vi "mfd_radio_bat.vi"() -> ()   [LabVIEW 2023]
uses:
  <vilib>/Utility/miscctls.llb/LVBoundsTypeDef.ctl
panel:
  in  "MFD_RcControl":T1
  in  "stop":bool
  out "MFD_RadioBattery":picture
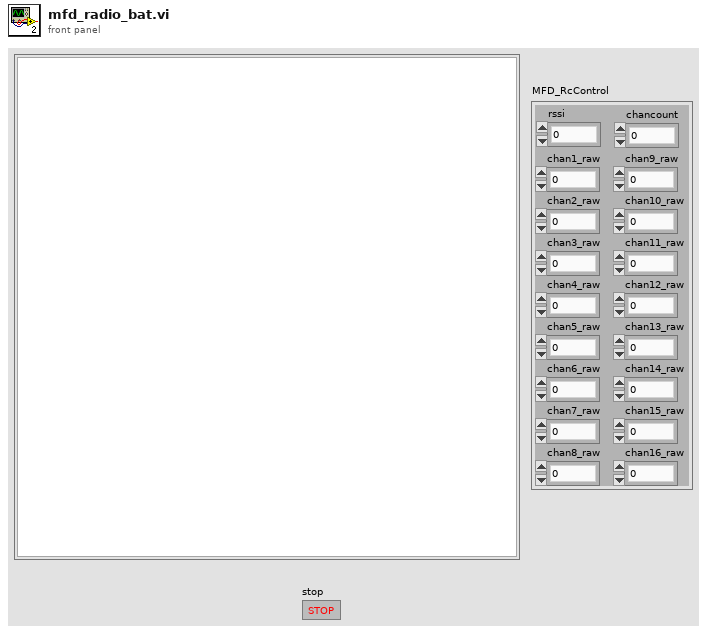
[diagram p1: front panel]
types:
  T1 = cluster{"chancount":u8, "chan1_raw":u16, "chan2_raw":u16, "chan3_raw":u16, "chan4_raw":u16, "chan5_raw":u16, "chan6_raw":u16, "chan7_raw":u16, "chan8_raw":u16, "chan9_raw":u16, "chan10_raw":u16, "chan11_raw":u16, "chan12_raw":u16, "chan13_raw":u16, "chan14_raw":u16, "chan15_raw":u16, "chan16_raw":u16, "rssi":u8}
  T2 = typedef "LVBoundsTypeDef.ctl" = cluster{"Width":u32, "Height":u32}
  T3 = cluster{"Width":u16, "Style":enum32{"Solid", "Dash", "Dot", "DashDot", "DashDotDot"}}
  T4 = cluster{"left":i16, "top":i16, "right":i16, "bottom":i16}
  T5 = cluster{"Font Name:":string, "Size":i16, "Strikeout?":bool, "Italic?":bool, "Underline?":bool, "Outline?":bool, "Shadow?":bool, "Bold?":bool}
  T6 = cluster{"horizontal":enum16{"left", "center", "right"}, "vertical":enum16{"top", "center", "bottom"}}
  T7 = enum16{"User-specified Font", "Application Font", "System Font", "Dialog Font"}
  T8 = cluster{"chancount":bool, "chan1_raw":bool, "chan2_raw":bool, "chan3_raw":bool, "chan4_raw":bool, "chan5_raw":bool, "chan6_raw":bool, "chan7_raw":bool, "chan8_raw":bool, "chan9_raw":bool, "chan10_raw":bool, "chan11_raw":bool, "chan12_raw":bool, "chan13_raw":bool, "chan14_raw":bool, "chan15_raw":bool, "chan16_raw":bool, "rssi":bool}
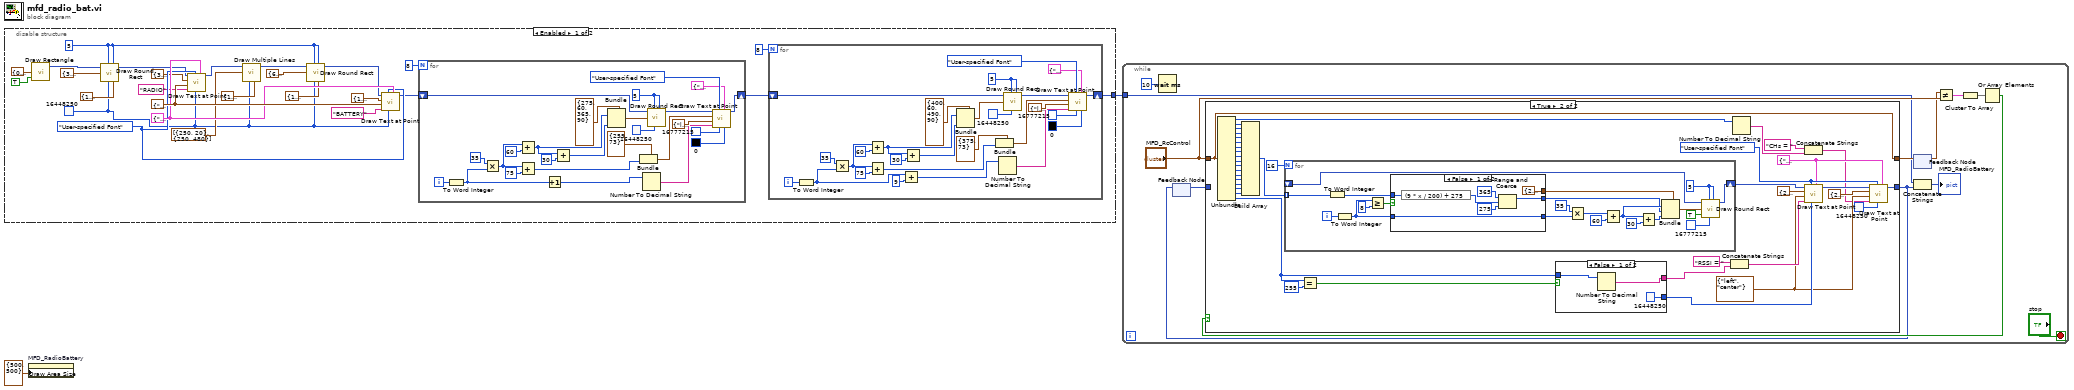
[diagram p0: block diagram]
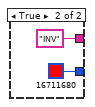
[diagram p4: hidden frame]
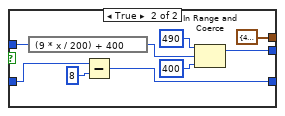
[diagram p5: hidden frame]
diagram:
  n1 = disable-structure shown="Enabled" {
    disable-tunnel: [w5 _] -> w1
    frame Enabled {
      w23 = T5 {"Font Name:"="r", "Size"=25, "Strikeout?"=FALSE, "Italic?"=FALSE, "Underline?"=FALSE, "Outline?"=FALSE, "Shadow?"=FALSE, "Bold?"=TRUE} ("[user-specified font]")
      w9 = u32 16448250 ("text color(black)")
      w22 = T7."User-specified Font" ("desired font(Application)")
      w24 = T6 {"horizontal"=enum."center", "vertical"=enum."top"} ("alignment(left, top)")
      w8 = i16 5 ("oval height")
      n2 = call <vilib>:"Draw Rectangle.vi"("rect"=T4 {"left"=0, "top"=0, "right"=500, "bottom"=500}, "fill?(F)"=TRUE) -> ("new picture"=w27:picture)  [unwired: 7 in]
      n3 = call <vilib>:"Draw Round Rect.vi"("picture"=w27, "oval width"=w8, "rect"=T4 {"left"=334, "top"=19, "right"=413, "bottom"=48}, "color(black)"=w9, "oval height"=w8, "pen"=T3 {"Width"=1, "Style"=enum."Solid"}) -> ("new picture"=w19:picture)  [unwired: 3 in]
      n4 = call <vilib>:"Draw Text at Point.vi"("[user-specified font]"=w23, "text color(black)"=w9, "desired font(Application)"=w22, "text"="RADIO", "alignment(left, top)"=w24, "origin"=cluster{"x":i16, "y":i16} {"x"=375, "y"=22}, "picture"=w19) -> ("new picture"=w18:picture)  [unwired: 3 in, 1 out]
      n5 = call <vilib>:"Draw Multiple Lines.vi"("picture"=w18, "line endpoints"=cluster{"x":i16, "y":i16}[] [{"x"=250, "y"=20}, {"x"=250, "y"=480}], "color(black)"=w9, "pen"=T3 {"Width"=1, "Style"=enum."Solid"} ("pen 2")) -> ("new picture"=w15:picture)  [unwired: 5 in]
      n6 = call <vilib>:"Draw Round Rect.vi"("picture"=w15, "oval width"=w8, "rect"=T4 {"left"=68, "top"=19, "right"=181, "bottom"=48} ("rect 4"), "color(black)"=w9, "oval height"=w8, "pen"=T3 {"Width"=1, "Style"=enum."Solid"}) -> ("new picture"=w10:picture)  [unwired: 3 in]
      n7 = call <vilib>:"Draw Text at Point.vi"("[user-specified font]"=w23, "text color(black)"=w9, "desired font(Application)"=w22, "text"="BATTERY", "alignment(left, top)"=w24, "origin"=cluster{"x":i16, "y":i16} {"x"=125, "y"=22} ("origin 2"), "picture"=w10) -> ("new picture"=w3:picture)  [unwired: 3 in, 1 out]
      n8 = for {
        N: 8 -> [_]
        shift-right: [w65] -> w4
        shift-left: w3 -> [w80]
        i -> [w77]
        w82 = i16 5 ("oval width")
        n9 = To Word Integer(number=w77) -> (16bit integer=w63:i16)
        n10 = Multiply(x=i16 35, y=w63) -> (x*y=w60:i16)
        n11 = Add(x=w60, y=i16 60) -> (x+y=w72:i16)
        n12 = Add(x=w60, y=i16 75) -> (x+y=w57:i16)
        n13 = Increment(x=w63) -> (x+1=w64:i16)
        n14 = Add(x=w72, y=i16 30 ("x")) -> (x+y=w74:i16)
        n15 = Bundle(cluster=T4 {"left"=275, "top"=60, "right"=365, "bottom"=90} ("rect"), "top"=w72, "bottom"=w74) -> (w78:T4)  [unwired: 2 in]
        n16 = Bundle(cluster=cluster{"x":i16, "y":i16} {"x"=259, "y"=73} ("origin"), "y"=w57) -> (w58:cluster{"x":i16, "y":i16})  [unwired: 1 in]
        n17 = Number To Decimal String(number=w64) -> (decimal integer string=w62:string)  [unwired: 1 in]
        n18 = call <vilib>:"Draw Round Rect.vi"("picture"=w80, "oval width"=w82, "rect"=w78, "color(black)"=u32 16448250, "oval height"=w82) -> ("new picture"=w66:picture)  [unwired: 4 in]
        n19 = call <vilib>:"Draw Text at Point.vi"("BG color(transparent)"=u32 0, "[user-specified font]"=T5 {"Font Name:"="channels", "Size"=18, "Strikeout?"=FALSE, "Italic?"=FALSE, "Underline?"=FALSE, "Outline?"=FALSE, "Shadow?"=FALSE, "Bold?"=TRUE}, "text color(black)"=u32 16777215, "desired font(Application)"=T7."User-specified Font", "text"=w62, "alignment(left, top)"=T6 {"horizontal"=enum."left", "vertical"=enum."center"}, "origin"=w58, "picture"=w66) -> ("new picture"=w65:picture)  [unwired: 2 in, 1 out]
      }
      n20 = for {
        N: 8 -> [_]
        shift-right: [w40] -> w5
        shift-left: w4 -> [w54]
        i -> [w52]
        w56 = i16 5 ("oval width")
        n21 = To Word Integer(number=w52) -> (16bit integer=w32:i16)
        n22 = Multiply(x=i16 35, y=w32) -> (x*y=w37:i16)
        n23 = Add(x=w37, y=i16 60) -> (x+y=w47:i16)
        n24 = Add(x=w37, y=i16 75) -> (x+y=w35:i16)
        n25 = Add(x=w32, y=i16 9) -> (x+y=w31:i16)
        n26 = Add(x=w47, y=i16 30 ("x")) -> (x+y=w49:i16)
        n27 = Bundle(cluster=T4 {"left"=400, "top"=60, "right"=490, "bottom"=90} ("rect 2"), "top"=w47, "bottom"=w49) -> (w53:T4)  [unwired: 2 in]
        n28 = Bundle(cluster=cluster{"x":i16, "y":i16} {"x"=375, "y"=73} ("origin"), "y"=w35) -> (w36:cluster{"x":i16, "y":i16})  [unwired: 1 in]
        n29 = Number To Decimal String(number=w31) -> (decimal integer string=w39:string)  [unwired: 1 in]
        n30 = call <vilib>:"Draw Round Rect.vi"("picture"=w54, "oval width"=w56, "rect"=w53, "color(black)"=u32 16448250, "oval height"=w56) -> ("new picture"=w41:picture)  [unwired: 4 in]
        n31 = call <vilib>:"Draw Text at Point.vi"("BG color(transparent)"=u32 0, "[user-specified font]"=T5 {"Font Name:"="channels", "Size"=18, "Strikeout?"=FALSE, "Italic?"=FALSE, "Underline?"=FALSE, "Outline?"=FALSE, "Shadow?"=FALSE, "Bold?"=TRUE}, "text color(black)"=u32 16777215, "desired font(Application)"=T7."User-specified Font", "text"=w39, "alignment(left, top)"=T6 {"horizontal"=enum."left", "vertical"=enum."center"}, "origin"=w36, "picture"=w41) -> ("new picture"=w40:picture)  [unwired: 2 in, 1 out]
      }
    }
    frame Disabled {
    }
  }
  n32 = property on="MFD_RadioBattery" class="Pict"("Draw Area Size"=T2 {"Width"=500, "Height"=500}) -> ()  [unwired: 2 in, 2 out]
  n33 = while {
    tunnel: w1 -> [w85]
    stop <- "stop" stop-if-true
    n34 = Wait (ms)(milliseconds to wait=u32 10) -> ()  [unwired: 1 out]
    n35 = feedback #1() -> (w92:picture)  [unwired: 1 in]
    n36 = feedback #2() -> (w86:T1)  [unwired: 1 in]
    n37 = Not Equal?(x=w86, y="MFD_RcControl") -> (x != y?=w90:T8)
    n38 = Cluster To Array(cluster=w90) -> (array=w89:bool[])
    n39 = Or Array Elements(Boolean array=w89) -> (logical OR=w88:bool)
    n40 = case shown="True" w88 {
      tunnel: "MFD_RcControl" -> [w95 w115]
      tunnel: [w96 w116] -> w84
      tunnel: w92 -> [w96 _]
      tunnel: [w95 w115] -> w87
      frame False {
      }
      frame True {
        w122 = T6 {"horizontal"=enum."left", "vertical"=enum."center"} ("alignment(left, top)")
        w123 = T5 {"Font Name:"="channels", "Size"=18, "Strikeout?"=FALSE, "Italic?"=FALSE, "Underline?"=FALSE, "Outline?"=FALSE, "Shadow?"=FALSE, "Bold?"=TRUE} ("[user-specified font]")
        w124 = T7."User-specified Font" ("desired font(Application)")
        n41 = Unbundle(w115) -> ("chancount"=w114:u8, "chan1_raw"=w113:u16, "chan2_raw"=w112:u16, "chan3_raw"=w111:u16, "chan4_raw"=w110:u16, "chan5_raw"=w109:u16, "chan6_raw"=w108:u16, "chan7_raw"=w107:u16, "chan8_raw"=w106:u16, "chan9_raw"=w105:u16, "chan10_raw"=w104:u16, "chan11_raw"=w103:u16, "chan12_raw"=w102:u16, "chan13_raw"=w101:u16, "chan14_raw"=w100:u16, "chan15_raw"=w99:u16, "chan16_raw"=w98:u16, "rssi"=w97:u8)
        n42 = Build Array(w113, w112, w111, w110, w109, w108, w107, w106, w105, w104, w103, w102, w101, w100, w99, w98) -> (w135:u16[])
        n43 = for {
          N: 16 -> [_]
          shift-right: [w141] -> w133
          shift-left: _ -> [w154]
          tunnel: w135 -> [w150] mode=indexing
          i -> [w152]
          w155 = i16 5 ("oval width")
          n44 = To Word Integer(number=w150) -> (16bit integer=w145:i16)
          n45 = To Word Integer(number=w152) -> (16bit integer=w144:i16)
          n46 = Greater Or Equal?(x=w144, y=i16 8) -> (x >= y?=w147:bool)
          n47 = case shown="False" w147 {
            tunnel: [T4 {"left"=275, "top"=60, "right"=365, "bottom"=90} ("rect") T4 {"left"=400, "top"=60, "right"=490, "bottom"=90} ("rect 2")] -> w146
            tunnel: w145 -> [w168 w177]
            tunnel: w144 -> [w167 w175]
            tunnel: [w167 w174] -> w143
            tunnel: [w163 w170] -> w142
            frame False {
              n48 = expression code="(9 * x / 200) + 275"(w168) -> (w165:i16)
              n49 = In Range and Coerce(upper limit=i16 365, x=w165, lower limit=i16 275) -> (coerced(x)=w163:i16)  [unwired: 1 out]
            }
            frame True {
              n50 = expression code="(9 * x / 200) + 400"(w177) -> (w171:i16)
              n51 = Subtract(x=w175, y=i16 8) -> (x-y=w174:i16)
              n52 = In Range and Coerce(upper limit=i16 490, x=w171, lower limit=i16 400) -> (coerced(x)=w170:i16)  [unwired: 1 out]
            }
          }
          n53 = Multiply(x=i16 35, y=w143) -> (x*y=w149:i16)
          n54 = Add(x=w149, y=i16 60) -> (x+y=w161:i16)
          n55 = Add(x=w161, y=i16 30 ("x")) -> (x+y=w160:i16)
          n56 = Bundle(cluster=w146, "top"=w161, "right"=w142, "bottom"=w160) -> (w153:T4)  [unwired: 1 in]
          n57 = call <vilib>:"Draw Round Rect.vi"("picture"=w154, "oval width"=w155, "rect"=w153, "fill?(F)"=TRUE, "color(black)"=u32 16777215, "oval height"=w155) -> ("new picture"=w141:picture)  [unwired: 3 in]
        }
        n58 = Equal?(x=w97, y=u8 255) -> (x = y?=w128:bool)
        n59 = case shown="False" w128 {
          tunnel: w97 -> [w138 _]
          tunnel: [w137 "INV"] -> w127
          tunnel: [u32 16448250 ("text color(black)") u32 16711680 ("text color(black)")] -> w126
          frame False {
            n60 = Number To Decimal String(number=w138) -> (decimal integer string=w137:string)  [unwired: 1 in]
          }
          frame True {
          }
        }
        n61 = Concatenate Strings("RSSI = " ("text"), w127) -> (w130:string)
        n62 = Number To Decimal String(number=w114) -> (decimal integer string=w118:string)  [unwired: 1 in]
        n63 = Concatenate Strings("CHs = " ("text"), w118) -> (w119:string)
        n64 = call <vilib>:"Draw Text at Point.vi"("[user-specified font]"=w123, "text color(black)"=w126, "desired font(Application)"=w124, "text"=w130, "alignment(left, top)"=w122, "origin"=cluster{"x":i16, "y":i16} {"x"=265, "y"=362}, "picture"=w133) -> ("new picture"=w125:picture)  [unwired: 3 in, 1 out]
        n65 = call <vilib>:"Draw Text at Point.vi"("[user-specified font]"=w123, "text color(black)"=u32 16448250, "desired font(Application)"=w124, "text"=w119, "alignment(left, top)"=w122, "origin"=cluster{"x":i16, "y":i16} {"x"=265, "y"=392} ("origin 2"), "picture"=w125) -> ("new picture"=w116:picture)  [unwired: 3 in, 1 out]
      }
    }
    n66 = feedback-in #1(w84) -> ()
    n67 = feedback-in #2(w87) -> ()
    n68 = Concatenate Strings(w85, w84) -> (→"MFD_RadioBattery":picture)
  }
